vi "visco.vi"(8 "min":dbl, 9 "max":dbl, 10 "input":dbl) -> (2 "output":dbl)   [LabVIEW 2015]
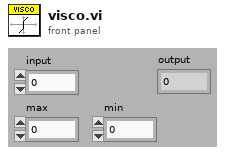
[diagram p1: front panel]
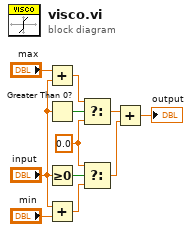
[diagram p0: block diagram]
diagram:
  w8 = 0.0 ("f")
  n1 = Add(x="max", y="input") -> (x+y=w10:dbl)
  n2 = Greater Than 0?(x="input") -> (x > 0?=w11:bool)
  n3 = Greater Or Equal To 0?(x="input") -> (x >= 0?=w2:bool)
  n4 = Add(x="input", y="min") -> (x+y=w1:dbl)
  n5 = Select(t=w10, s=w11, f=w8) -> (s? t:f=w7:dbl)
  n6 = Select(t=w8, s=w2, f=w1) -> (s? t:f=w6:dbl)
  n7 = Add(x=w7, y=w6) -> (x+y=→"output":dbl)
